vi "Autonomous.vi"() -> ()   [LabVIEW 2019]
doc: "This VI starts when autonomous period begins, and will automatically be terminated when it ends. You can carry out timed or sensor driven operations directly to I/O or to subsystems without needing to return to the caller."
uses:
  Motion_Profiler_Class-master/MotionProfiles.lvclass
  <vilib>/Rock Robotics/WPI/SafetyOutput/WPI_SafetyOutputConfigMenu.ctl
  <vilib>/Rock Robotics/Network Tables/NT Read String.vi
  <vilib>/Rock Robotics/WPI/Utilities/WPI_GetSetVariantRefNum.vi
  <vilib>/Utility/file.llb/Read Delimited Spreadsheet (string).vi
  <vilib>/Utility/file.llb/Read Delimited Spreadsheet (DBL).vi
panel:
  out "MotionProfiles out":refnum<class "MotionProfiles.lvclass">
  out "Left Motor":T1(graph)
  out "Left Throttle":dbl(graph)
  out "Right Motor":T2(graph)
  out "Right Throttle":dbl(graph)
  out "Right Bottom Buf Count":i32
  out "Left Bottom Buf Count":i32
  out "Right Under Run":bool
  out "Left Under Run":bool
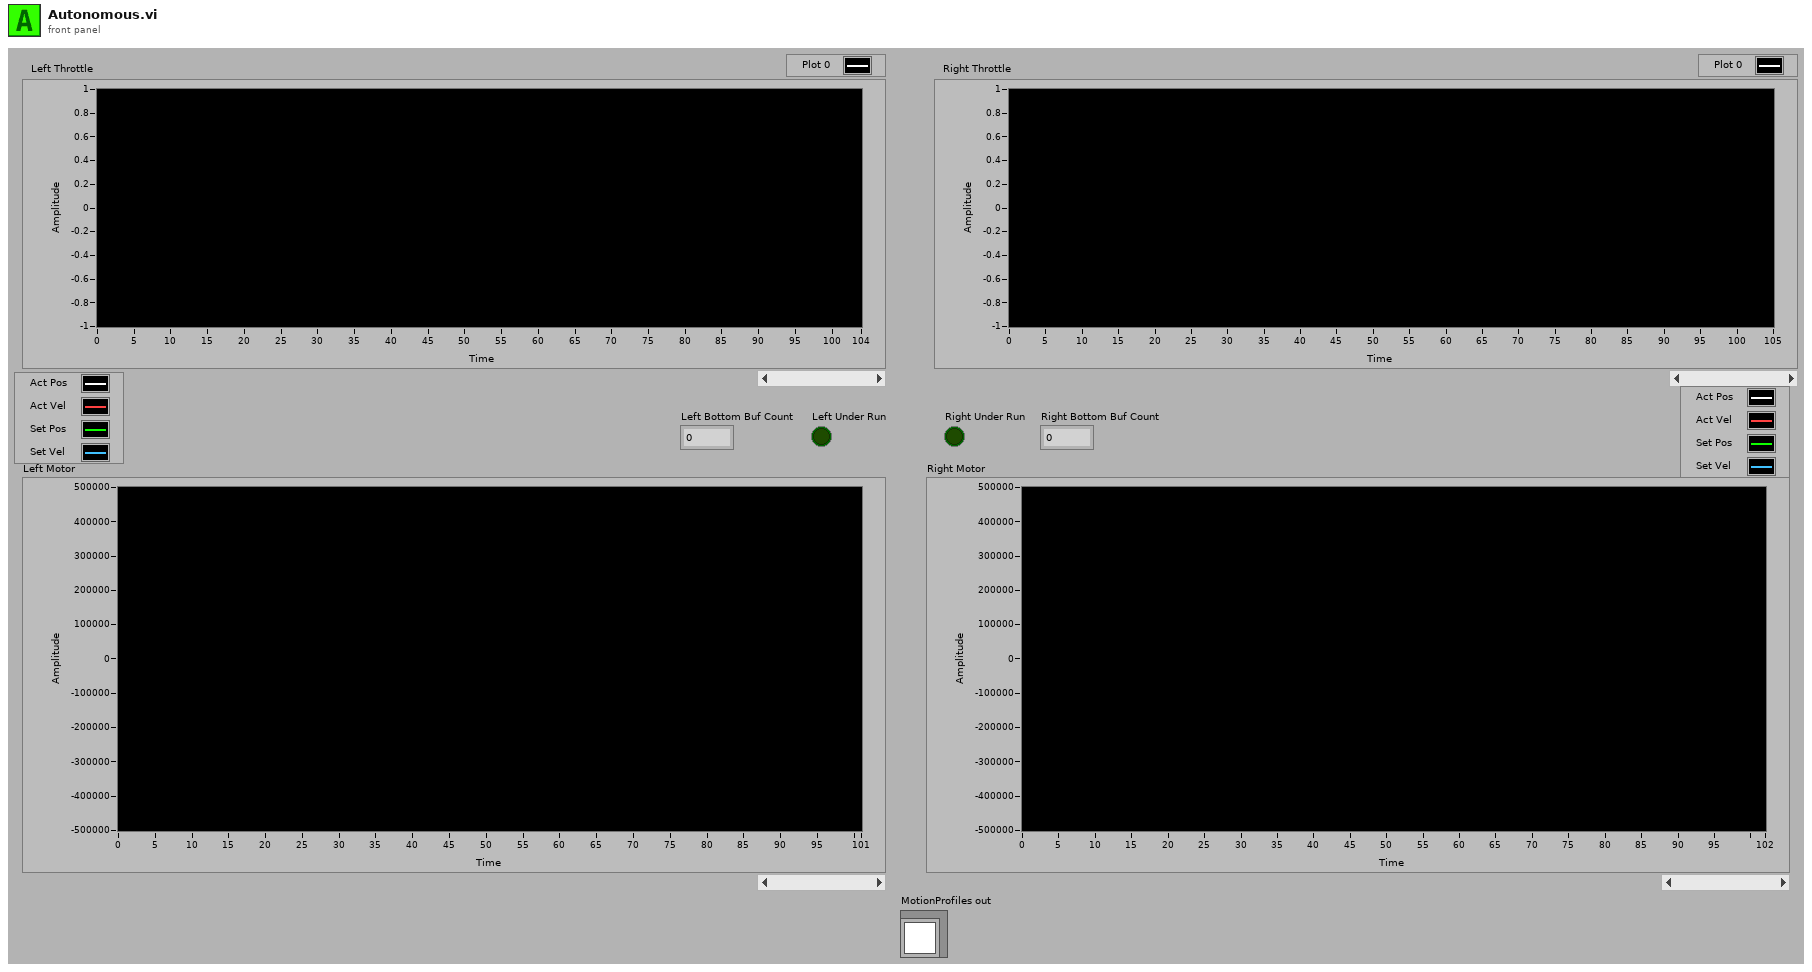
[diagram p1: front panel]
types:
  T1 = cluster{"Set_Pos_(u)":i32, "Set_Pos_(u)":i32, "Act_Vel_(u/100ms)":i32, "Set_Vel_(u/100ms)":i32}
  T2 = cluster{"Set_Vel_(u/100ms)":i32, "Act_Vel_(u/100ms)":i32, "Set_Pos_(u)":i32, "Act_Pos(u)":i32}
  T3 = typedef "WPI_SafetyOutputConfigMenu.ctl" = enum16{"Enable", "Disable"}
  T4 = typedef "WPI_RobotDriveDevRef.ctl" = cluster{"DevStatus":errorcluster, "Motors[]":T5[], "Square Inputs":bool, "Max Output":dbl}
  T5 = typedef "WPI_MotorControlDeviceRef.ctl" = cluster{"DeviceStatus":errorcluster, "Type":T6, "PWM":cluster{"PWM Channel":T7, "DeadBand":T8}, "CAN":cluster{"Device Number":u8, "SetOutput VI Ref":variant, "GetOutput VI Ref":variant, "Enable VI Ref":variant, "Disable VI Ref":variant, "Data":variant}, "Invert":bool, "DIO PWM":cluster{"PWM \"Enable\" Channel":T7, "DIOChannel":T9, "PWM Rate":dbl}}
  T6 = typedef "WPI_MotorControlType.ctl" = enum16{"PWM", "CAN", "DIO PWM"}
  T7 = typedef "FPGA_DIOPWMChannel.ctl" = enum8{"PWM 0", "PWM 1", "PWM 2", "PWM 3", "PWM 4", "PWM 5", "PWM 6", "PWM 7", "PWM 8", "PWM 9", "PWM MXP 0", "PWM MXP 1", "PWM MXP 2", "PWM MXP 3", "PWM MXP 4", "PWM MXP 5", "PWM MXP 6", "PWM MXP 7", "PWM MXP 8", "PWM MXP 9", "Invalid"}
  T8 = typedef "WPI_PWMDeadband.ctl" = cluster{"Name":string, "maxPositivePwm":i32, "minPositivePwm":i32, "centerPwm":i32, "maxNegativePwm":i32, "minNegativePwm":i32, "angularRange":u16}
  T9 = typedef "FPGA_DIOChannel.ctl" = enum8{"DIO 0", "DIO 1", "DIO 2", "DIO 3", "DIO 4", "DIO 5", "DIO 6", "DIO 7", "DIO 8", "DIO 9", "DIO MXP 0", "DIO MXP 1", "DIO MXP 2", "DIO MXP 3", "DIO MXP 4", "DIO MXP 5", "DIO MXP 6", "DIO MXP 7", "DIO MXP 8", "DIO MXP 9", "DIO MXP 10", "DIO MXP 11", "DIO MXP 12", "DIO MXP 13", "DIO MXP 14", "DIO MXP 15", "SPI Port CS1", "SPI Port CS2", "SPI Port CS3", "SPI Port MISO", "SPI Port MOSI", "Invalid"}
  T10 = typedef "MotionProfiles.lvclass/MotionProfile_MP_Class_Status.ctl" = cluster{"Motion Profile Status":cluster{"Top Buffer Remaining":i32, "Top Buffer Count":i32, "Bottom Buffer Count":i32, "Has Underrun?":bool, "Is Underrun?":bool, "Active Point Valid?":bool, "Is Last?":bool, "Profile Slot Select 0":i32, "Output Enable":i32, "Time Duration (ms)":i32, "Profile Slot Select 1":i32}, "TalonState":T11, "MP Is Done":bool, "MP Is Executing":bool, "Set_Vel_(u/100ms)":i32, "Set_Pos_(u)":i32, "Act_Vel_(u/100ms)":i32, "Act_Pos(u)":i32, "Throtle":dbl}
  T11 = typedef "MotionProfiles.lvclass/MotionProfile_TalonSetValueEnum.ctl" = enum16{"Disable", "Enable", "Hold"}
  T12 = enum16{"Pick Up Ball", "Pick Up Hatch", "Shoot Ball", "Shoot Hatch", "Low Ball", "Middle Ball", "High Ball", "High Hatch", "Middle Hatch", "Low Hatch", "Cargo Ball", "Ball Loading Station", "Ball Ground", "Reserve"}
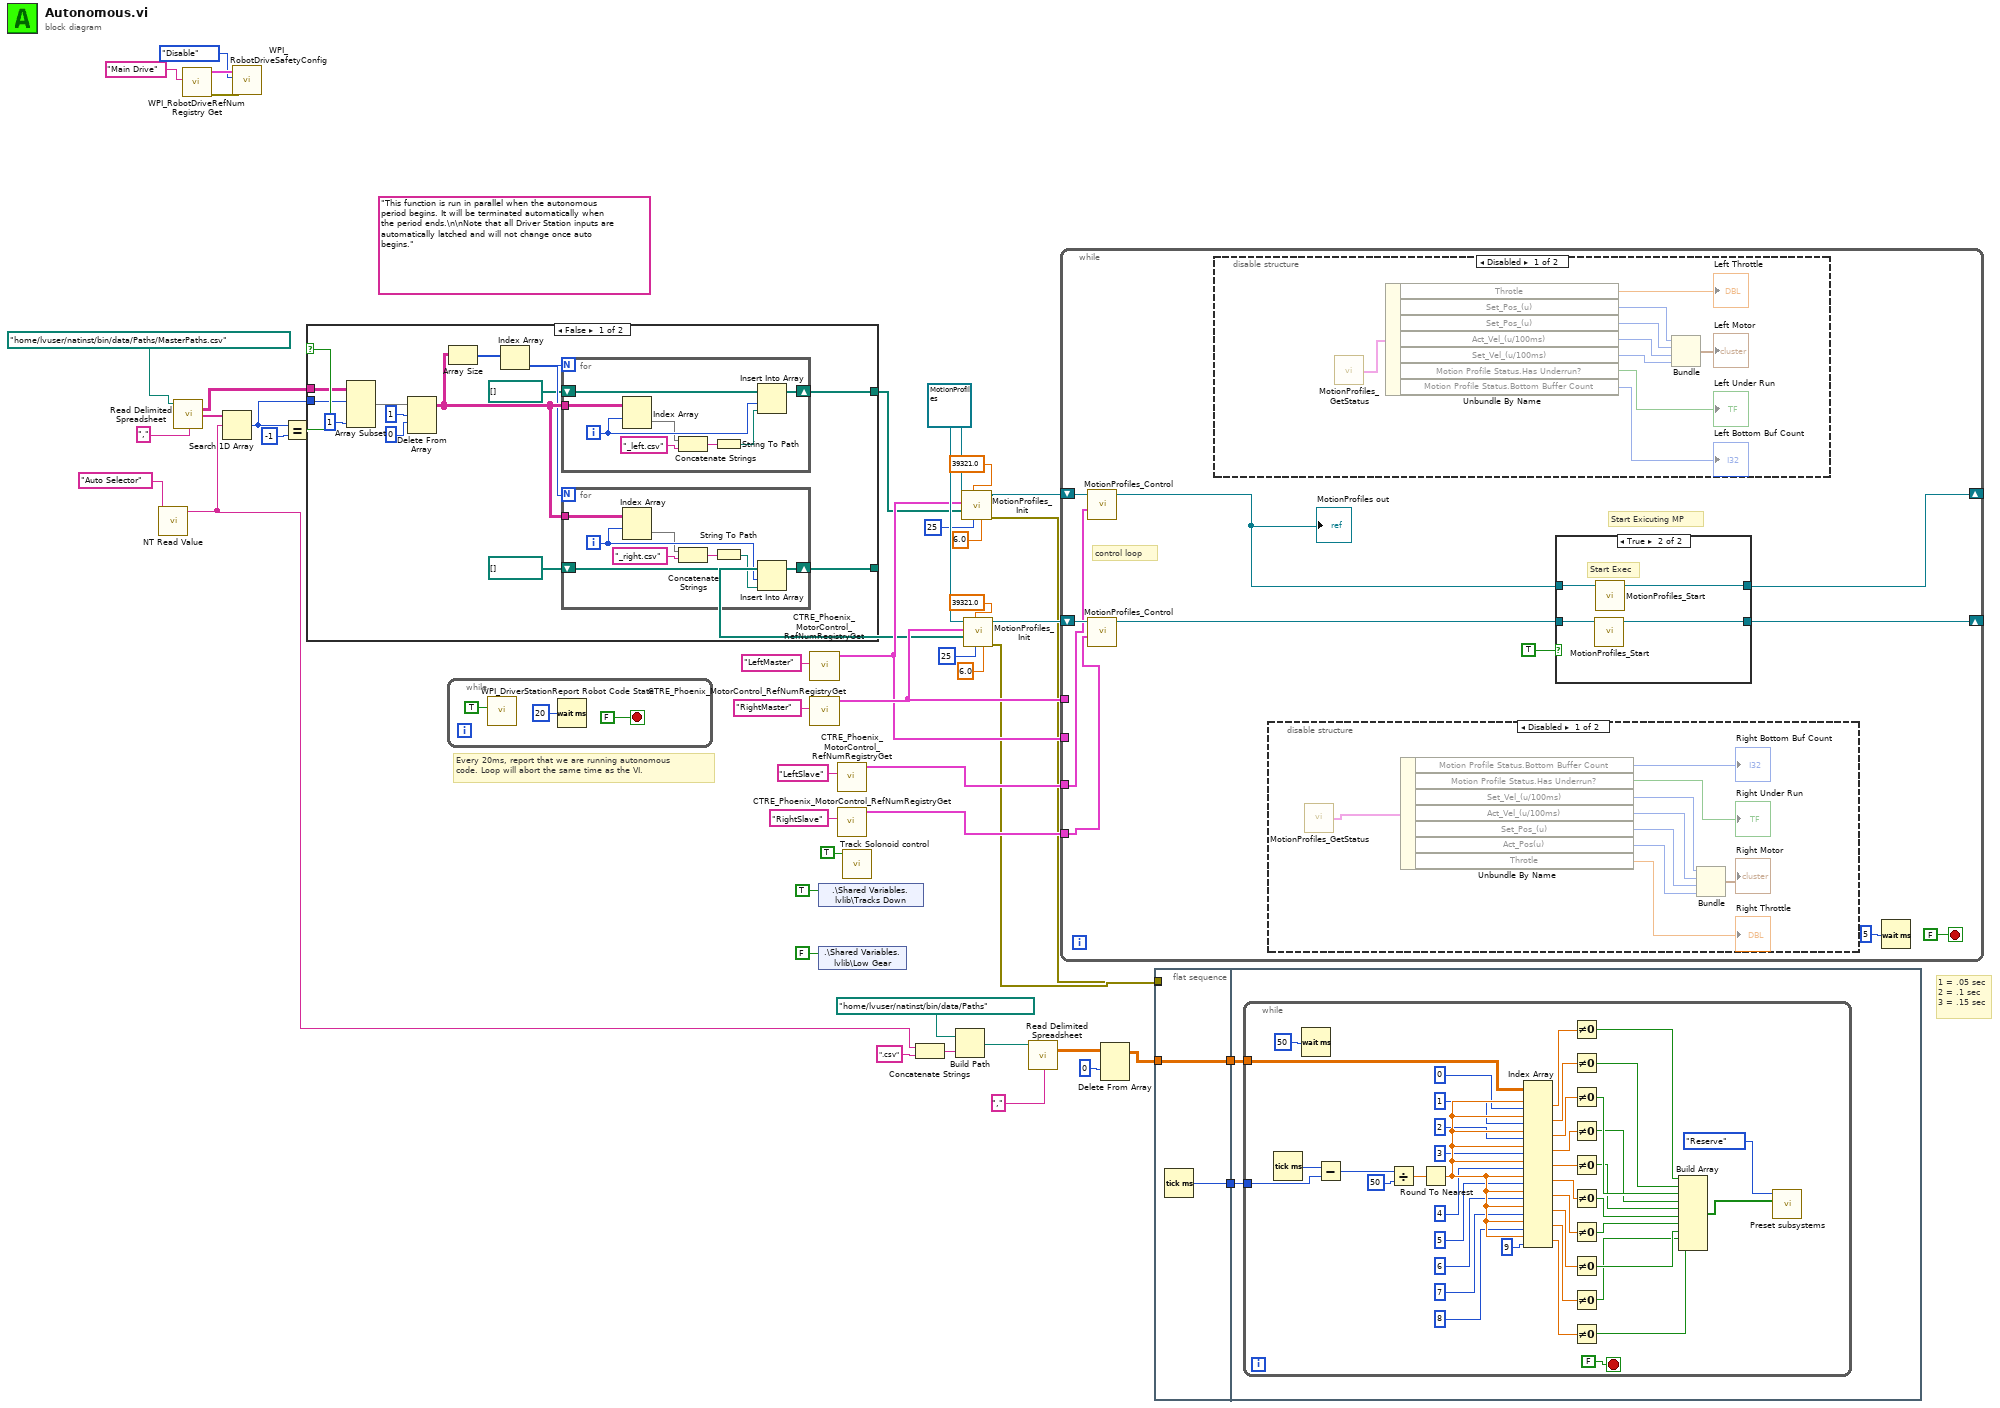
[diagram p0: block diagram]
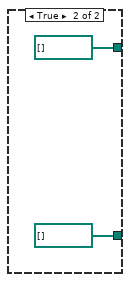
[diagram p2: hidden frame]
diagram:
  w41 = refnum<class "MotionProfiles.lvclass"> refnum ("MotionProfiles.lvclass")
  (unwired) "This function is run in parallel when the autonomous period begins. It will be terminated automatically when the period ends.\n\nNote that all Driver Station inputs are automatically latched and will not change once auto begins."
  # "1 = .05 sec\n2 = .1 sec\n3 = .15 sec"
  # "Every 20ms, report that we are running autonomous\ncode. Loop will abort the same time as the VI."
  n1 = call-poly <vilib>:"NT Read Value.vi"("Name"="Auto Selector") -> ("String"=w4:string)  [unwired: 9 in, 1 out]
  n2 = call-poly <vilib>:"Read Delimited Spreadsheet.vi"("file path (dialog if empty)"=path "/home/lvuser/natinst/bin/data/Paths/MasterPaths.csv" ("file path (use dialog)"), "delimiter (\\t)"="," ("delimiter (\\t)")) -> ("all rows"=w14:string[][], "first row"=w19:string[])  [unwired: 8 in, 4 out]
  n3 = call <vilib>:"WPI_RobotDriveRefNum Registry Get.vi"("refnum name"="Main Drive") -> ("error out"=w23:errorcluster, "RobotDriveDevRef"=w22:T4)  [unwired: 9 in]
  n4 = Search 1D Array(1D array=w19, element=w4) -> (index of element=w13:i32)  [unwired: 1 in]
  n5 = call <vilib>:"WPI_RobotDriveSafetyConfig.vi"("error in (no error)"=w23, "mode"=WPI_SafetyOutputConfigMenu."Disable", "RobotDriveDevRef"=w22) -> ()  [unwired: 7 in, 2 out]
  n6 = Equal?(x=w13, y=-1) -> (x = y?=w15:bool)
  n7 = case shown="False" w15 {
    tunnel: w14 -> [w60 _]
    tunnel: w13 -> [w59 _]
    tunnel: [w52 path[] [] ("CSV File Path")] -> w16
    tunnel: [w48 path[] [] ("CSV File Path")] -> w17
    frame False {
      n8 = Array Subset(array=w60, index (row)=w59, length (col)=1 ("length")) -> (w57:string[][])  [unwired: 2 in]
      n9 = Delete From Array(array=w57, length=1, index (row)=0) -> (array with subset deleted=w51:string[][])  [unwired: 1 in, 1 out]
      n10 = Array Size(array=w51) -> (size(s)=w53:i32[])
      n11 = Index Array(array=w53) -> (element=w50:i32)  [unwired: 1 in]
      n12 = for {
        N: w50 -> [_]
        shift-right: [w67] -> w48
        shift-left: path[] [] ("CSV File Path") -> [w68]
        tunnel: w51 -> [w65]
        i -> [w66]
        n13 = Index Array(array=w65, index (row)=w66) -> (element=w64:string[])  [unwired: 1 in]
        n14 = Concatenate Strings(w64, "_left.csv" ("string")) -> (w61:string)
        n15 = String To Path(string=w61) -> (path=w62:path)
        n16 = Insert Into Array(array=w68, index=w66, new element=w62) -> (w67:path[])
      }
      n17 = for {
        N: w50 -> [_]
        shift-right: [w74] -> w52
        shift-left: path[] [] ("CSV File Path") -> [w76]
        tunnel: w51 -> [w72]
        i -> [w73]
        n18 = Index Array(array=w72, index (row)=w73) -> (element=w70:string[])  [unwired: 1 in]
        n19 = Concatenate Strings(w70, "_right.csv" ("string")) -> (w69:string)
        n20 = String To Path(string=w69) -> (path=w75:path)
        n21 = Insert Into Array(array=w76, index=w73, new element=w75) -> (w74:path[])
      }
    }
    frame True {
    }
  }
  n22 = while {
    stop <- FALSE stop-if-true
    n23 = call <vilib>:"WPI_DriverStationReport Robot Code State.vi"("Autonomous"=TRUE) -> ()  [unwired: 10 in, 1 out]
    n24 = Wait (ms)(milliseconds to wait=u32 20) -> ()  [unwired: 1 out]
  }
  n25 = call <vilib>:"CTRE_Phoenix_MotorControl_RefNumRegistryGet.vi"("refnum name"="LeftMaster") -> ("PhoenixMotorControlDevRef"=w32:T5)  [unwired: 9 in, 1 out]
  n26 = call <vilib>:"CTRE_Phoenix_MotorControl_RefNumRegistryGet.vi"("refnum name"="RightMaster") -> ("PhoenixMotorControlDevRef"=w33:T5)  [unwired: 9 in, 1 out]
  n27 = shared-variable ".\\Shared Variables.lvlib\\Tracks Down"(TRUE ("High Gear")) -> ()  [unwired: 1 in, 1 out]
  n28 = shared-variable ".\\Shared Variables.lvlib\\Low Gear"(FALSE ("High Gear")) -> ()  [unwired: 1 in, 1 out]
  n29 = call <vilib>:"CTRE_Phoenix_MotorControl_RefNumRegistryGet.vi"("refnum name"="LeftSlave") -> ("PhoenixMotorControlDevRef"=w29:T5)  [unwired: 9 in, 1 out]
  n30 = call <vilib>:"CTRE_Phoenix_MotorControl_RefNumRegistryGet.vi"("refnum name"="RightSlave") -> ("PhoenixMotorControlDevRef"=w28:T5)  [unwired: 9 in, 1 out]
  n31 = call "Track Solonoid control.vi"("Manual Tracks"=TRUE) -> ()  [unwired: 11 in]
  n32 = Concatenate Strings(w4, ".csv" ("string")) -> (w9:string)
  n33 = Build Path(base path=path "/home/lvuser/natinst/bin/data/Paths" ("file path (use dialog)"), name or relative path=w9) -> (appended path=w7:path)
  n34 = call "MotionProfiles_Init.vi"("Wheel_Diameter (in)"=6.0 ("Wheel Diameter"), "MP_Frame_Rate_(ms)"=25, "Encoder_CPR_4x"=39321.0, "CSV File Path"=w17, "PhoenixMotorControlDevRef"=w32, "MotionProfiles in"=w41) -> ("error out"=w3:errorcluster, "MotionProfiles out"=w44:refnum<class "MotionProfiles.lvclass">)  [unwired: 4 in]
  n35 = call "MotionProfiles_Init.vi"("Wheel_Diameter (in)"=6.0, "MP_Frame_Rate_(ms)"=25, "Encoder_CPR_4x"=39321.0, "CSV File Path"=w16, "PhoenixMotorControlDevRef"=w33, "MotionProfiles in"=w41) -> ("error out"=w5:errorcluster, "MotionProfiles out"=w42:refnum<class "MotionProfiles.lvclass">)  [unwired: 4 in]
  n36 = call-poly <vilib>:"Read Delimited Spreadsheet.vi"("file path (dialog if empty)"=w7, "delimiter (\\t)"="," ("delimiter (\\t)")) -> ("all rows"=w10:dbl[][])  [unwired: 8 in, 5 out]
  n37 = while {
    shift-right: [w87] -> _
    shift-left: w44 -> [w90]
    shift-right: [w88] -> _
    shift-left: w42 -> [w89]
    tunnel: w33 -> [_]
    tunnel: w32 -> [_]
    tunnel: w29 -> [w85]
    tunnel: w28 -> [w84]
    stop <- FALSE stop-if-true
    # "control loop"
    # "Start Exicuting MP"
    n38 = call "MotionProfiles_Control.vi"("PhoenixMotorControlDevRef Slave"=w85, "MotionProfiles in"=w90) -> ("MotionProfiles out"=w82:refnum<class "MotionProfiles.lvclass">)  [unwired: 8 in, 1 out]
    "MotionProfiles out" <- w82
    n39 = call "MotionProfiles_Control.vi"("PhoenixMotorControlDevRef Slave"=w84, "MotionProfiles in"=w89) -> ("MotionProfiles out"=w83:refnum<class "MotionProfiles.lvclass">)  [unwired: 8 in, 1 out]
    n40 = disable-structure shown="Disabled" {
      frame Disabled {
        n41 = call "MotionProfiles_GetStatus.vi"() -> ("MP_Class_Status"=w110:T10)  [unwired: 13 in, 2 out]
        n42 = Unbundle By Name(w110) -> ("Throtle"=→"Left Throttle":dbl, "Set_Pos_(u)"=w103:i32, "Set_Pos_(u)"=w104:i32, "Act_Vel_(u/100ms)"=w105:i32, "Set_Vel_(u/100ms)"=w106:i32, "Motion Profile Status.Has Underrun?"=→"Left Under Run":bool, "Motion Profile Status.Bottom Buffer Count"=→"Left Bottom Buf Count":i32)
        n43 = Bundle("Set_Pos_(u)"=w103, "Set_Pos_(u)"=w104, "Act_Vel_(u/100ms)"=w105, "Set_Vel_(u/100ms)"=w106) -> (→"Left Motor":T1)  [unwired: 1 in]
      }
      frame Enabled {
      }
    }
    n44 = disable-structure shown="Disabled" {
      frame Disabled {
        n45 = call "MotionProfiles_GetStatus.vi"() -> ("MP_Class_Status"=w101:T10)  [unwired: 13 in, 2 out]
        n46 = Unbundle By Name(w101) -> ("Motion Profile Status.Bottom Buffer Count"=→"Right Bottom Buf Count":i32, "Motion Profile Status.Has Underrun?"=→"Right Under Run":bool, "Set_Vel_(u/100ms)"=w97:i32, "Act_Vel_(u/100ms)"=w96:i32, "Set_Pos_(u)"=w95:i32, "Act_Pos(u)"=w94:i32, "Throtle"=→"Right Throttle":dbl)
        n47 = Bundle("Set_Vel_(u/100ms)"=w97, "Act_Vel_(u/100ms)"=w96, "Set_Pos_(u)"=w95, "Act_Pos(u)"=w94) -> (→"Right Motor":T2)  [unwired: 1 in]
      }
      frame Enabled {
      }
    }
    n48 = case shown="True" TRUE {
      tunnel: w82 -> [w112 w116]
      tunnel: w83 -> [w111 w114]
      tunnel: [w111 w113] -> w88
      tunnel: [w112 w115] -> w87
      frame False {
      }
      frame True {
        # "Start Exec"
        n49 = call "MotionProfiles_Start.vi"("MotionProfiles in"=w114) -> ("MotionProfiles out"=w113:refnum<class "MotionProfiles.lvclass">)  [unwired: 9 in, 1 out]
        n50 = call "MotionProfiles_Start.vi"("MotionProfiles in"=w116) -> ("MotionProfiles out"=w115:refnum<class "MotionProfiles.lvclass">)  [unwired: 9 in, 1 out]
      }
    }
    n51 = Wait (ms)(milliseconds to wait=u32 5) -> ()  [unwired: 1 out]
  }
  n52 = Delete From Array(array=w10, index (row)=0) -> (array with subset deleted=w6:dbl[][])  [unwired: 2 in, 1 out]
  n53 = flat-sequence {
    tunnel: [w118] -> w47
    tunnel: w6 -> [w117]
    tunnel: [w117] -> w46
    tunnel: w5 -> [_]
    tunnel: w3 -> [_]
    tunnel: w47 -> [w120]
    tunnel: w46 -> [w119]
    frame #0 {
      n54 = Tick Count (ms)() -> (millisecond timer value=w118:u32)
    }
    frame #1 {
      n55 = while {
        tunnel: w120 -> [w158]
        tunnel: w119 -> [w154]
        stop <- FALSE stop-if-true
        n56 = Tick Count (ms)() -> (millisecond timer value=w160:u32)
        n57 = Wait (ms)(milliseconds to wait=u32 50) -> ()  [unwired: 1 out]
        n58 = Subtract(x=w160, y=w158) -> (x-y=w156:u32)
        n59 = Divide(x=w156, y=u32 50) -> (x/y=w159:dbl)
        n60 = Round To Nearest(number=w159) -> (nearest integer value=w153:dbl)
        n61 = Index Array(array=w154, index (row) #1=w153, index (col) #1=0 ("disabled index (col)"), index (row) #2=w153, index (col) #2=1 ("disabled index (col)"), index (row) #3=w153, index (col) #3=2 ("disabled index (col)"), index (row) #4=w153, index (col) #4=3 ("disabled index (col)"), index (row) #5=w153, index (col) #5=4 ("disabled index (col)"), index (row) #6=w153, index (col) #6=5 ("disabled index (col)"), index (row) #7=w153, index (col) #7=6 ("disabled index (col)"), index (row) #8=w153, index (col) #8=7 ("disabled index (col)"), index (row) #9=w153, index (col) #9=8 ("disabled index (col)"), index (row) #10=w153, index (col) #10=9 ("disabled index (col)")) -> (element #1=w152:dbl, element #2=w151:dbl, element #3=w150:dbl, element #4=w149:dbl, element #5=w148:dbl, element #6=w147:dbl, element #7=w146:dbl, element #8=w145:dbl, element #9=w144:dbl, element #10=w143:dbl)
        n62 = Not Equal To 0?(x=w152) -> (x != 0?=w131:bool)
        n63 = Not Equal To 0?(x=w151) -> (x != 0?=w130:bool)
        n64 = Not Equal To 0?(x=w150) -> (x != 0?=w129:bool)
        n65 = Not Equal To 0?(x=w149) -> (x != 0?=w128:bool)
        n66 = Not Equal To 0?(x=w148) -> (x != 0?=w127:bool)
        n67 = Not Equal To 0?(x=w147) -> (x != 0?=w126:bool)
        n68 = Not Equal To 0?(x=w146) -> (x != 0?=w125:bool)
        n69 = Not Equal To 0?(x=w145) -> (x != 0?=w124:bool)
        n70 = Not Equal To 0?(x=w144) -> (x != 0?=w123:bool)
        n71 = Not Equal To 0?(x=w143) -> (x != 0?=w122:bool)
        n72 = Build Array(w131, w130, w129, w128, w127, w126, w125, w124, w123, w122) -> (w121:bool[])
        n73 = call "Preset subsystems.vi"("appended array"=w121, "Enum"=T12."Reserve") -> ()  [unwired: 10 in]
      }
    }
  }
